vi "getFlags.vi"(11 "PUBREL in":refnum<class "PUBREL.lvclass">) -> (0 "RETAIN":bool, 1 "QoS":T1, 2 "DUP":bool, 3 "PUBREL out":refnum<class "PUBREL.lvclass">)   [LabVIEW 2013, in "MQTT_Control_Packets.lvlib" / "PUBREL.lvclass"]
uses:
  PUBREL.lvclass
  ControlPacket/QualityOfService -- enum.ctl
  ControlPacket/ControlPacket.lvclass
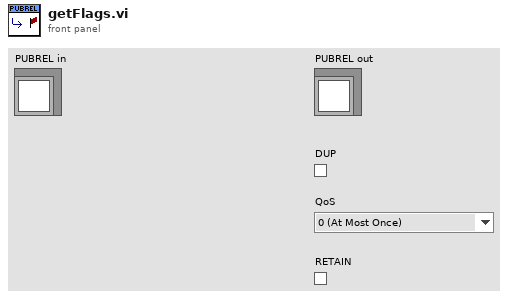
[diagram p1: front panel]
types:
  T1 = typedef "MQTT_Control_Packets.lvlib/ControlPacket.lvclass/QualityOfService -- enum.ctl" = enum16{"0 (At Most Once)", "1 (At Least Once)", "2 (Exactly Once)"}
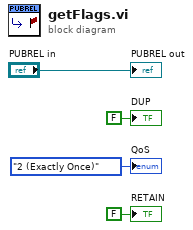
[diagram p0: block diagram]
diagram:
  "PUBREL out" <- "PUBREL in"
  "QoS" <- QualityOfService_--_enum."2 (Exactly Once)" ("QoS")
  "DUP" <- FALSE ("DUP")
  "RETAIN" <- FALSE ("RETAIN")
